vi "Read Mux Routes.vi"(8 "error in (no error)":errorcluster, 11 "Mux in":refnum<class "Mux.lvclass">) -> (0 "error out":errorcluster, 2 "Current Routes":i32[](array[numeric]), 3 "Mux out":refnum<class "Mux.lvclass">)   [LabVIEW 2022 SP3, in "VideoMux.lvlib" / "Mux.lvclass"]
uses:
  Mux.lvclass
  Mux.lvclass/Mux.ctl
  <vilib>/IlluminatedG/lv-stream/stream/Stream.lvclass/Stream.ctl
  <vilib>/IlluminatedG/lv-stream/stream/Dispatch Sniffer Data.vi
  <vilib>/IlluminatedG/lv-stream/stream/Prepared.vi
  <vilib>/IlluminatedG/lv-stream/Endpoint/Cast Sniffer Callback.vi
  <vilib>/Utility/error.llb/Error Cluster From Error Code.vi
  <vilib>/IlluminatedG/lv-stream/stream/Stream.lvclass
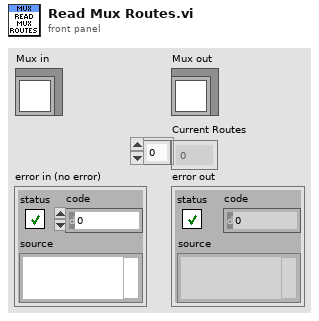
[diagram p1: front panel]
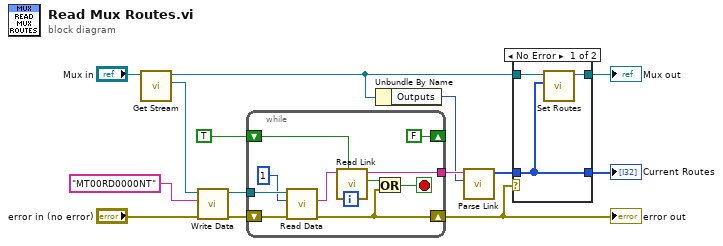
[diagram p0: block diagram]
diagram:
  n1 = call "Get Stream.vi"("Mux in"="Mux in") -> ("Stream"=w7:refnum<class "Stream.lvclass">, "Mux out"=w2:refnum<class "Mux.lvclass">)  [unwired: 8 in, 1 out]
  n2 = call <vilib>:"Write Data.vi"("error in (no error)"="error in (no error)", "Data"="MT00RD0000NT", "Stream in"=w7) -> ("error out"=w9:errorcluster, "Stream out"=w10:refnum<class "Stream.lvclass">)  [unwired: 7 in]
  n3 = while {
    tunnel: w10 -> [w19]
    shift-right: [FALSE] -> _
    shift-left: TRUE -> [w24]
    shift-right: [w15] -> w3
    shift-left: w9 -> [w18]
    tunnel: [w21] -> w13
    stop <- w22 stop-if-true
    n4 = call <vilib>:"Read Data.vi"("error in (no error)"=w18, "Count"=1 ("byte count"), "Stream in"=w19) -> ("error out"=w15:errorcluster, "Data"=w16:string)  [unwired: 6 in, 1 out]
    n5 = call "Read Link.vi"("Reset? (F)"=w24, "Input"=w16) -> ("End?"=w23:bool, "Full Output"=w21:string)  [unwired: 8 in]
    n6 = Or(x=w23, y=w15) -> (x .or. y?=w22:bool)
  }
  "error out" <- w3
  n7 = Unbundle By Name(w2) -> ("Outputs"=w1:i32)
  n8 = call "Parse Link.vi"("Outputs (All)"=w1, "String"=w13) -> ("Routes"=w12:i32[])  [unwired: 9 in]
  n9 = case shown="No Error" w3 {
    tunnel: w12 -> [w26 _]
    tunnel: [w27 w28] -> w6
    tunnel: [w26 _] -> w5
    tunnel: w2 -> [w25 w28]
    frame No Error {
      n10 = call "Set Routes.vi"("Routes"=w26, "Mux in"=w25) -> ("Mux out"=w27:refnum<class "Mux.lvclass">)  [unwired: 8 in, 1 out]
    }
    frame Error {
    }
  }
  "Mux out" <- w6
  "Current Routes" <- w5
